vi "get version string.vi"(8 "error in (no error)":errorcluster, 10 "buffer_len":u64, 11 "version_out":string) -> (0 "error out":errorcluster, 2 "function return":u32(ring), 3 "version_out out":string)   [LabVIEW 2023, in "uhd.lvlib"]
doc: "UHD_API uhd_error uhd_get_version_string(char* version_out, size_t buffer_len);"
uses:
  <userlib>/uhd/uhd.lvlib
  <userlib>/uhd/uhd.dll
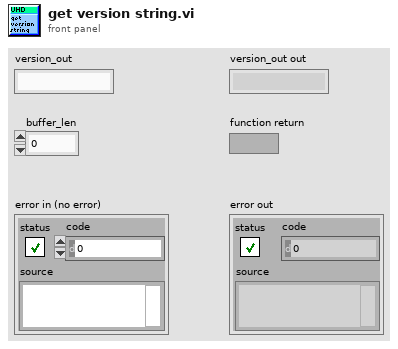
[diagram p1: front panel]
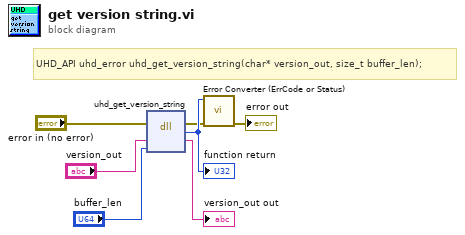
[diagram p0: block diagram]
diagram:
  # "UHD_API uhd_error uhd_get_version_string(char* version_out, size_t buffer_len);"
  n1 = dll-call lib="C:/Program Files/National Instruments/LabVIEW 2023/user.lib/uhd/uhd.*" fn="uhd_get_version_string"(error in="error in (no error)", "version_out"="version_out", "buffer_len"="buffer_len") -> (error out=w2:errorcluster, w7:u32, "version_out"=→"version_out out":string)  [unwired: 3 in, 1 out]
  "function return" <- w7
  n2 = call <userlib>:"Error Converter (ErrCode or Status).vi"("error in (no error)"=w2, "error code"=w7) -> ("error out"=→"error out":errorcluster)  [unwired: 9 in]
